vi "TMP35.vi"(7 "Analog Ref Override":dbl, 8 "Error In":errorcluster, 10 "Analog Channel":u8, 11 "LINX Resource":T1) -> (0 "Error Out":errorcluster, 2 "Temp C":dbl, 3 "LINX Resource":T1)   [LabVIEW 2014, in "LMH-LINX.lvlib" / "TMP3x.lvlib"]
doc: "Read temperature from TMP35"
uses:
  TMP3x.lvlib
  Private/Type Defs/LINX Ref.ctl
  Private/Type Defs/Platform.ctl
  Private/Type Defs/Interface.ctl
  Private/Device/Type Defs/LINX Device Config.ctl
  Private/Device/Type Defs/TCP Config.ctl
  Private/Device/Type Defs/Channels.ctl
  Peripherals/Analog/Analog Read 1 Chan.vi
  Peripherals/Analog/Analog Read N Chans.vi
  Private/Local IO/LinxAnalogRead.vi
  Utilities/Check Channel.vi
  Private/Utilties/Generate Error.vi
  LMH-LINX.lvlib
  Private/Device/Device.lvlib
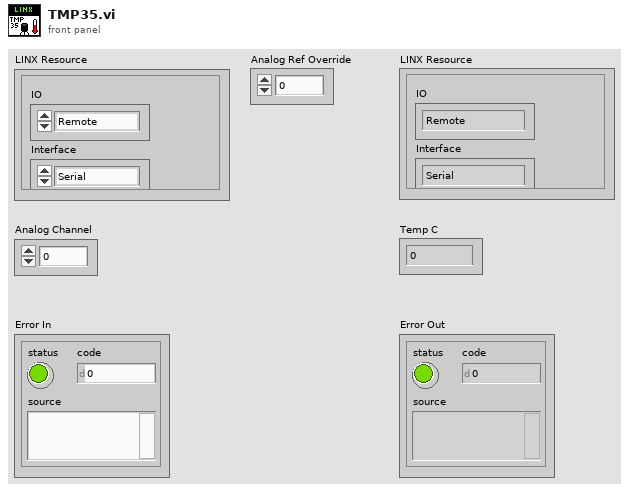
[diagram p1: front panel]
types:
  T1 = typedef "LMH-LINX.lvlib/LINX Ref.ctl" = cluster{"IO":T2, "Interface":T3, "LINX Device Config":T4}
  T2 = typedef "LMH-LINX.lvlib/Platform.ctl" = enum16{"Remote", "Local"}
  T3 = typedef "LMH-LINX.lvlib/Interface.ctl" = enum16{"Serial", "TCP"}
  T4 = typedef "LMH-LINX.lvlib/Device.lvlib/LINX Device Config.ctl" = cluster{"Interface":T3, "COM Port":refnum<visa-resource-name>, "TCP Configuration":T5, "Device Family":u8, "Device ID":u8, "Device Name":string, "TCP Ref":refnum<k5>, "Channels":T6}
  T5 = typedef "LMH-LINX.lvlib/Device.lvlib/TCP Config.ctl" = cluster{"IP Address":string, "Port":u16}
  T6 = typedef "LMH-LINX.lvlib/Channels.ctl" = cluster{"DI":u8[], "DO":u8[], "AI":u8[], "AO":u8[], "PWM":u8[], "QE":u8[], "UART":u8[], "I2C 2":u8[], "SPI":u8[], "CAN":u8[], "Servo":u8[], "AI Ref (V)":dbl, "AI Resolution (Bits)":u8, "AO Ref (V)":dbl, "AO Resolution (Bits)":u8}
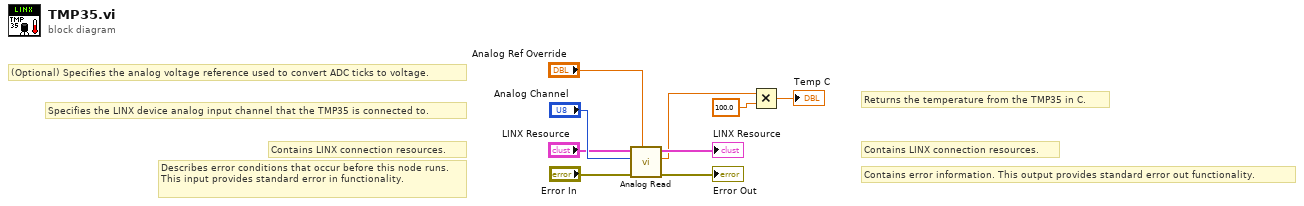
[diagram p0: block diagram]
diagram:
  # "Returns the temperature from the TMP35 in C."
  # "(Optional) Specifies the analog voltage reference used to convert ADC ticks to voltage."
  # "Specifies the LINX device analog input channel that the TMP35 is connected to."
  # "Contains LINX connection resources."
  # "Contains error information. This output provides standard error out functionality."
  # "Contains LINX connection resources."
  # "Describes error conditions that occur before this node runs. This input provides standard error in functionality."
  n1 = call-poly "Analog Read.vi"("Analog Ref Override (V)"="Analog Ref Override", "Error In"="Error In", "Analog Channel"="Analog Channel", "LINX Resource"="LINX Resource") -> ("Error Out"=→"Error Out":errorcluster, "Voltage"=w3:dbl, "LINX Resource"=→"LINX Resource":T1)  [unwired: 4 in, 1 out]
  n2 = Multiply(x=w3, y=100.0) -> (x*y=→"Temp C":dbl)
